vi "dataValueToXml.vi"(8 "error in (no error)":errorcluster, 11 "SingleTone in":refnum<class "SingleTone.lvclass">) -> (0 "error out":errorcluster, 2 "dataValueXml":refnum<class "xmlNode.lvclass">, 3 "SingleTone out":refnum<class "SingleTone.lvclass">)   [LabVIEW 2011, in "Tools.lvlib" / "Scripting.lvlib" / "SingleTone.lvclass"]
uses:
  SingleTone.lvclass
  xmlNode/xmlNode.lvclass
  SingleTone.lvclass/SingleTone.ctl
  DatabaseHelpers/Database Objects/Channel/Channel.lvclass
  ScriptEvent.lvclass
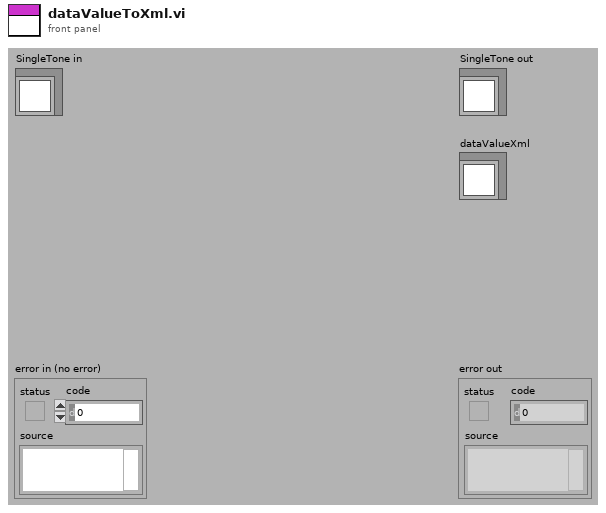
[diagram p1: front panel]
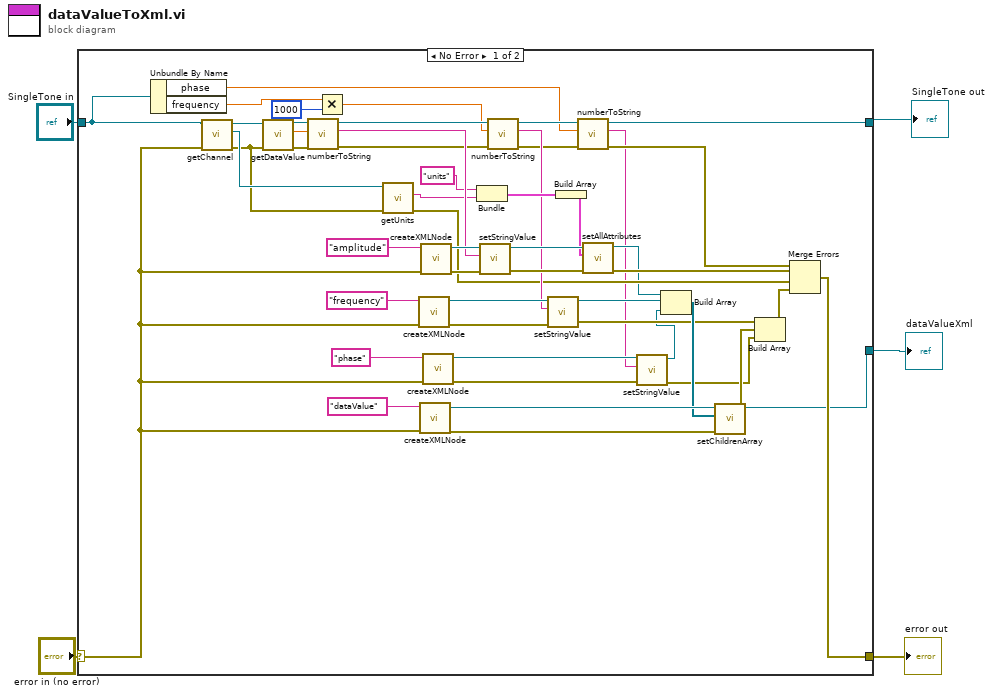
[diagram p0: block diagram]
diagram:
  n1 = case shown="No Error" "error in (no error)" {
    selector: "error in (no error)" -> [w15 w57]
    tunnel: [w9 w58] -> w2
    tunnel: "SingleTone in" -> [w13 w58]
    tunnel: [w22 w57] -> w4
    tunnel: [w21 _] -> w1
    frame No Error {
      n2 = Unbundle By Name(w13) -> ("phase"=w8:dbl, "frequency"=w36:dbl)
      n3 = call-dynamic "getChannel.vi"("error in (no error)"=w15, "ScriptEvent.lvclass in"=w13) -> ("error out"=w40:errorcluster, "Channel.lvclass"=w41:refnum<class "Channel.lvclass">, "ScriptEvent.lvclass out"=w44:refnum<class "SingleTone.lvclass">)  [unwired: 7 in]
      n4 = call "getDataValue.vi"("error in (no error)"=w40, "ScriptEvent.lvclass in"=w44) -> ("error out"=w43:errorcluster, "dataValue"=w42:dbl, "ScriptEvent.lvclass out"=w45:refnum<class "SingleTone.lvclass">)  [unwired: 7 in]
      n5 = call "numberToString.vi"("error in (no error)"=w43, "Numeric"=w42, "ScriptEvent in"=w45) -> ("error out"=w37:errorcluster, "String"=w53:string, "ScriptEvent out"=w38:refnum<class "SingleTone.lvclass">)  [unwired: 6 in]
      n6 = Multiply(x=w36, y=1000) -> (x*y=w20:dbl)
      n7 = call-dynamic "getUnits.vi"("error in (no error)"=w40, "Channel.lvclass in"=w41) -> ("error out"=w32:errorcluster, "units"=w50:string)  [unwired: 7 in, 1 out]
      n8 = call "createXMLNode.vi"("error in (no error)"=w15, "name"="frequency") -> ("error out"=w34:errorcluster, "xmlNode out"=w35:refnum<class "xmlNode.lvclass">)  [unwired: 8 in]
      n9 = call "createXMLNode.vi"("error in (no error)"=w15, "name"="dataValue") -> ("error out"=w26:errorcluster, "xmlNode out"=w30:refnum<class "xmlNode.lvclass">)  [unwired: 8 in]
      n10 = call "createXMLNode.vi"("error in (no error)"=w15, "name"="amplitude") -> ("error out"=w54:errorcluster, "xmlNode out"=w55:refnum<class "xmlNode.lvclass">)  [unwired: 8 in]
      n11 = call "createXMLNode.vi"("error in (no error)"=w15, "name"="phase") -> ("error out"=w16:errorcluster, "xmlNode out"=w17:refnum<class "xmlNode.lvclass">)  [unwired: 8 in]
      n12 = Bundle("units", "units"=w50) -> (w48:cluster{string, "units":string})  [unwired: 1 in]
      n13 = call-dynamic "setStringValue.vi"("error in (no error)"=w54, "stringValue"=w53, "xmlNode.lvclass in"=w55) -> ("error out"=w52:errorcluster, "xmlNode.lvclass out"=w51:refnum<class "xmlNode.lvclass">)  [unwired: 7 in]
      n14 = call "numberToString.vi"("error in (no error)"=w37, "Numeric"=w20, "ScriptEvent in"=w38) -> ("error out"=w11:errorcluster, "String"=w33:string, "ScriptEvent out"=w12:refnum<class "SingleTone.lvclass">)  [unwired: 6 in]
      n15 = call-dynamic "setStringValue.vi"("error in (no error)"=w34, "stringValue"=w33, "xmlNode.lvclass in"=w35) -> ("error out"=w25:errorcluster, "xmlNode.lvclass out"=w28:refnum<class "xmlNode.lvclass">)  [unwired: 7 in]
      n16 = Build Array(w48) -> (w47:cluster{string, "units":string}[])
      n17 = call "numberToString.vi"("error in (no error)"=w11, "Numeric"=w8, "ScriptEvent in"=w12) -> ("error out"=w10:errorcluster, "String"=w7:string, "ScriptEvent out"=w9:refnum<class "SingleTone.lvclass">)  [unwired: 6 in]
      n18 = call-dynamic "setAllAttributes.vi"("error in (no error)"=w52, "attributes"=w47, "xmlNode in"=w51) -> ("error out"=w46:errorcluster, "xmlNode out"=w29:refnum<class "xmlNode.lvclass">)  [unwired: 7 in]
      n19 = call-dynamic "setStringValue.vi"("error in (no error)"=w16, "stringValue"=w7, "xmlNode.lvclass in"=w17) -> ("error out"=w6:errorcluster, "xmlNode.lvclass out"=w14:refnum<class "xmlNode.lvclass">)  [unwired: 7 in]
      n20 = Build Array(w29, w28, w14) -> (w27:refnum<class "xmlNode.lvclass">[])
      n21 = call-dynamic "setChildrenArray.vi"("error in (no error)"=w26, "Children"=w27, "xmlNode.lvclass in"=w30) -> ("error out"=w24:errorcluster, "xmlNode.lvclass out"=w21:refnum<class "xmlNode.lvclass">)  [unwired: 7 in]
      n22 = Build Array(w25, w24, w6) -> (w23:errorcluster[])
      n23 = Merge Errors(w10, w46, w32, w23) -> (w22:errorcluster)
    }
    frame Error {
    }
  }
  "error out" <- w4
  "SingleTone out" <- w2
  "dataValueXml" <- w1
